vi "decide_where_to_move--trigonometric order.vi"(2 "tour_in_progress":T1[](array[typedef]), 3 "chessboard":T2[][](array[typedef])) -> (0 "square_to_move_forward_to":T1, 1 "action":T4)   [LabVIEW 2020, in "core.lvlib"]
uses:
  core.lvlib
  action.ctl
  core_data/chessboard_index.ctl
  core_data/chess_square.ctl
  core_data/neighbour_square.ctl
  pause (global variable).vi
  core_data/core_data.lvlib
panel:
  # "Development\ncontrols/indicators useful for development and testing, but which are not outputs of the VI"
  # "Input\nInputs to the VI"
  # "Output\nOutputs of the VI"
  # "Description\n\nBlank VI with error handling case. \n\nSummarize the use of this VI in this space."
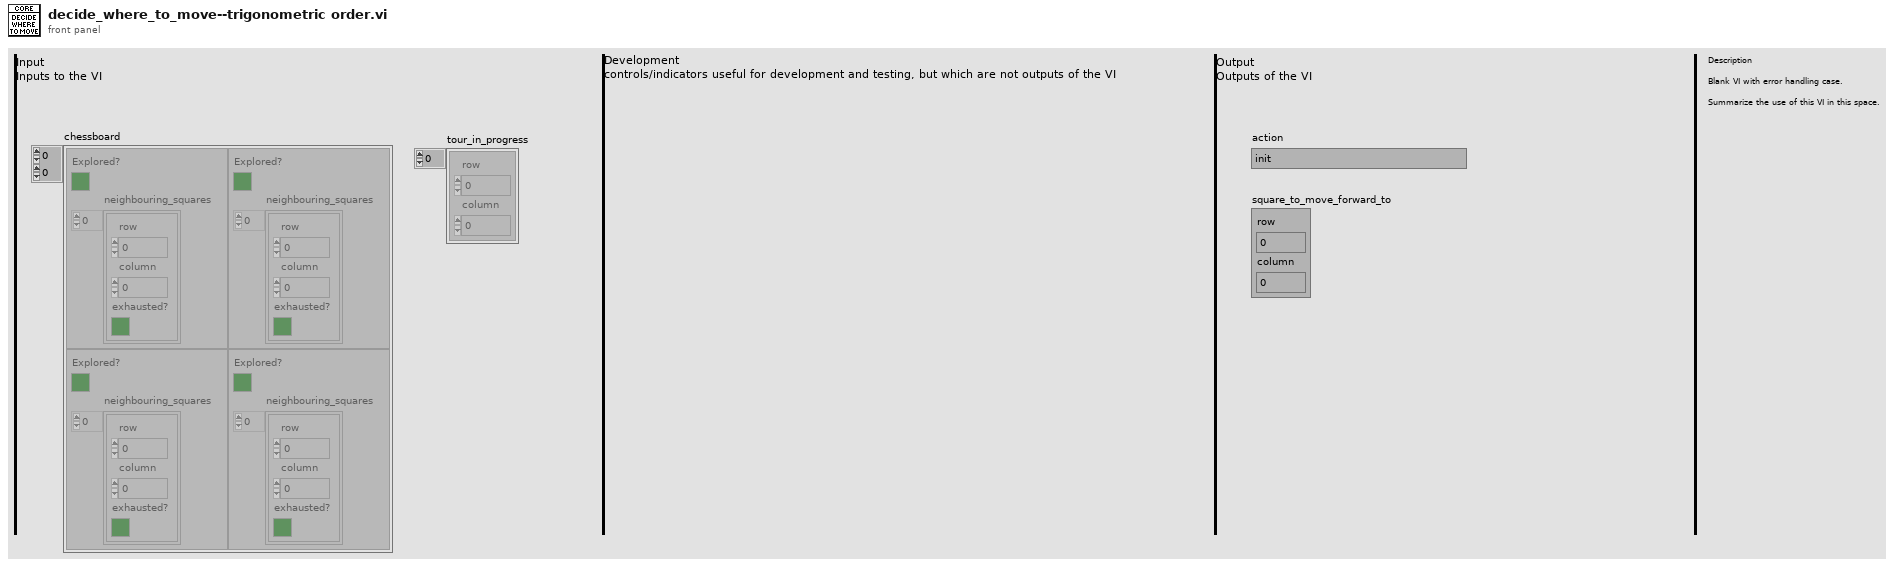
[diagram p1: front panel]
types:
  T1 = typedef "core.lvlib/core_data.lvlib/chessboard_index.ctl" = cluster{"row":u8, "column":u8}
  T2 = typedef "core.lvlib/core_data.lvlib/chess_square.ctl" = cluster{"Explored?":bool, "neighbouring_squares":T3[]}
  T3 = typedef "core.lvlib/core_data.lvlib/neighbour_square.ctl" = cluster{"row":u8, "column":u8, "exhausted?":bool}
  T4 = typedef "core.lvlib/action.ctl" = enum16{"init", "move_forward", "move_backward", "complete_tour", "exit", "be idle (do nothing)"}
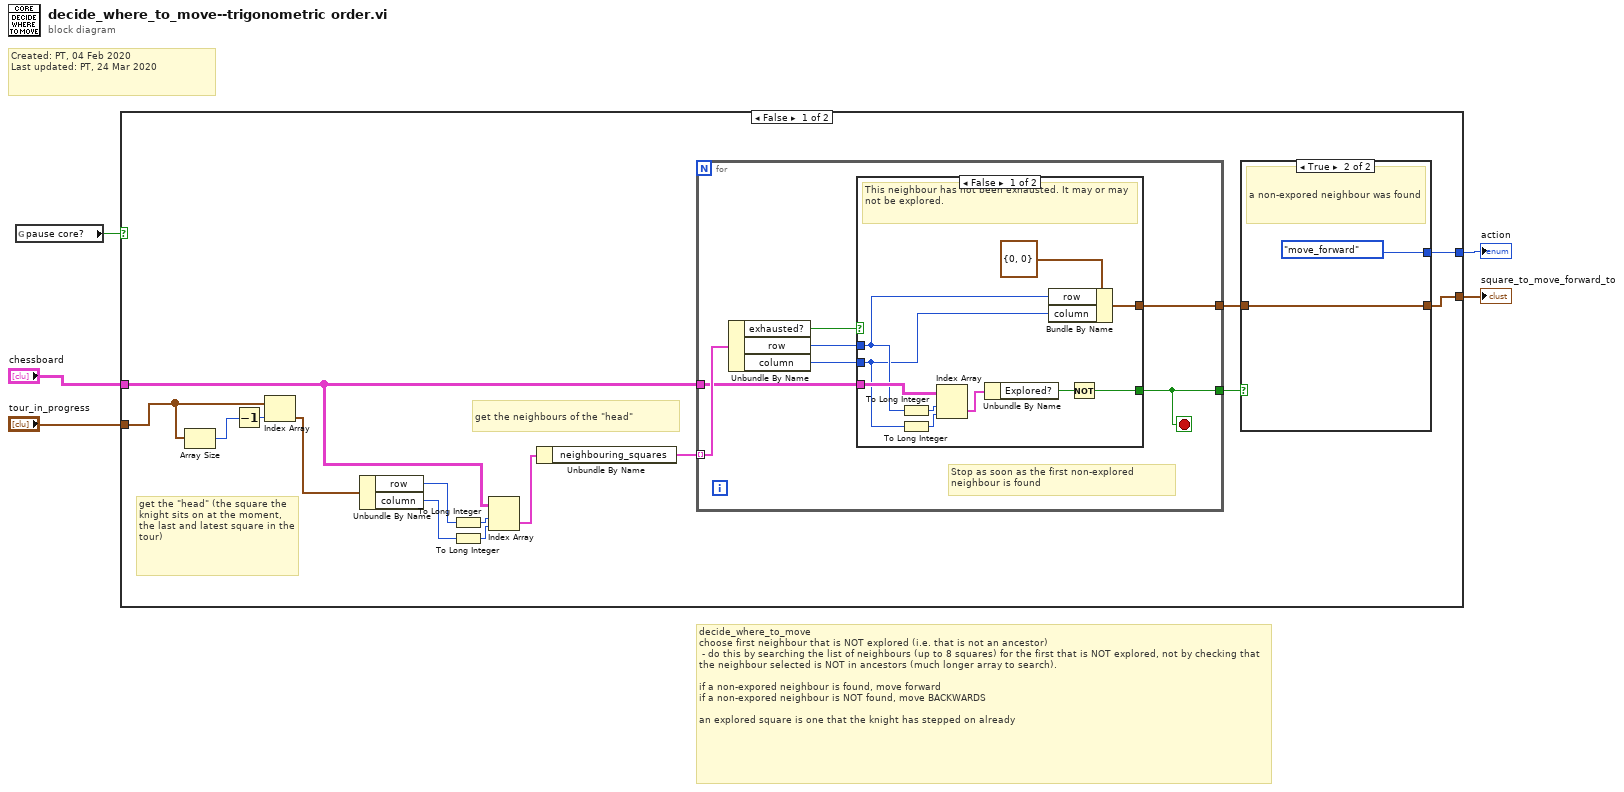
[diagram p0: block diagram]
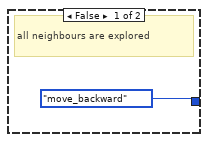
[diagram p2: hidden frame]
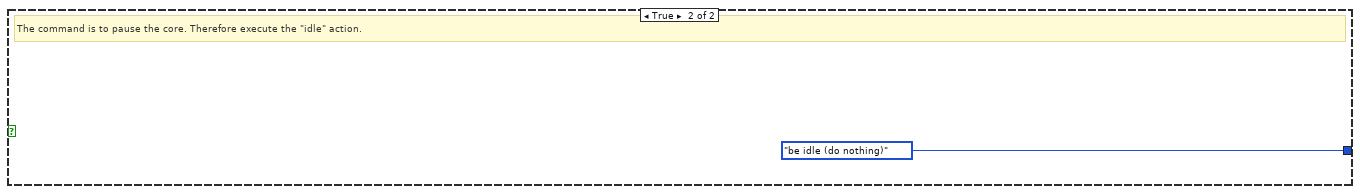
[diagram p4: hidden frame]
diagram:
  # "decide_where_to_move\nchoose first neighbour that is NOT explored (i.e. that is not an ancestor)\n - do this by searching the list of neighbours (up to 8 squares) for the first that is NOT explored, not by checking that the neighbour selected is NOT in ancestors (much longer array to search).\n\nif a non-expored neighbour is found, move forward\nif a non-expored neighbour is NOT found, move BACKWARDS\n\nan explored square is one that the knight has stepped on already"
  # "Created: PT, 04 Feb 2020\nLast updated: PT, 24 Mar 2020"
  n1 = global read "pause (global variable).vi" "pause core?"() -> (w3:bool)
  n2 = case shown="False" w3 {
    tunnel: [w20 action."be idle (do nothing)" ("action")] -> w5
    tunnel: [w16 _] -> w4
    tunnel: "chessboard" -> [w11 _]
    tunnel: "tour_in_progress" -> [w12 _]
    frame False {
      # "get the neighbours of the \"head\""
      # "get the \"head\" (the square the knight sits on at the moment, the last and latest square in the tour)"
      n3 = Array Size(array=w12) -> (size(s)=w13:i32)
      n4 = Decrement(x=w13) -> (x-1=w14:i32)
      n5 = Index Array(array=w12, index=w14) -> (element=w15:T1)
      n6 = Unbundle By Name(w15) -> ("row"=w9:u8, "column"=w8:u8)
      n7 = To Long Integer(number=w9) -> (32bit integer=w7:i32)
      n8 = To Long Integer(number=w8) -> (32bit integer=w6:i32)
      n9 = Index Array(array=w11, index (row)=w7, index (col)=w6) -> (element=w10:T2)
      n10 = Unbundle By Name(w10) -> ("neighbouring_squares"=w19:T3[])
      n11 = for {
        tunnel: w19 -> [w29] mode=indexing
        tunnel: w11 -> [w28]
        tunnel: [w25] -> w18
        tunnel: [w24] -> w17
        stop <- w25 stop-if-true
        # "Stop as soon as the first non-explored neighbour is found"
        n12 = Unbundle By Name(w29) -> ("exhausted?"=w30:bool, "row"=w27:u8, "column"=w26:u8)
        n13 = case shown="False" w30 {
          tunnel: w28 -> [w34 _]
          tunnel: w27 -> [w32 _]
          tunnel: w26 -> [w31 _]
          tunnel: [w39 _] -> w25
          tunnel: [w37 _] -> w24
          frame False {
            # "This neighbour has not been exhausted. It may or may not be explored."
            n14 = To Long Integer(number=w32) -> (32bit integer=w36:i32)
            n15 = To Long Integer(number=w31) -> (32bit integer=w35:i32)
            n16 = Index Array(array=w34, index (row)=w36, index (col)=w35) -> (element=w33:T2)
            n17 = Unbundle By Name(w33) -> ("Explored?"=w40:bool)
            n18 = Bundle By Name(cluster=T1 {"row"=0, "column"=0} ("square_to_move_forward_to"), "row"=w32, "column"=w31) -> (w37:T1)
            n19 = Not(x=w40) -> (.not. x?=w39:bool)
          }
          frame True {
            # "A neighbour that is exhausted is, implicitly, one that has been explored."
          }
        }
      }
      n20 = case shown="True" w18 {
        tunnel: [action."move_backward" ("action") action."move_forward" ("action")] -> w20
        tunnel: w17 -> [_ w22]
        tunnel: [_ w22] -> w16
        frame False {
          # "all neighbours are explored"
        }
        frame True {
          # "a non-expored neighbour was found"
        }
      }
    }
    frame True {
      # "The command is to pause the core. Therefore execute the \"idle\" action."
    }
  }
  "action" <- w5
  "square_to_move_forward_to" <- w4
